vi "Define Test.vi"(8 "error in":errorcluster, 11 "Label (VI Title)":string) -> (0 "error out":errorcluster, 2 "Properties.Test":refnum<class "Properties.Test.lvclass">)   [LabVIEW 2021, in "Bananas.lvlib"]
uses:
  Bananas.lvlib
  <vilib>/addons/_JKI Toolkits/Caraya/classes/Properties.Test/Properties.Test.lvclass
  <vilib>/addons/_JKI Toolkits/Caraya/classes/Test/Test.lvclass
  Banana/Banana.lvclass
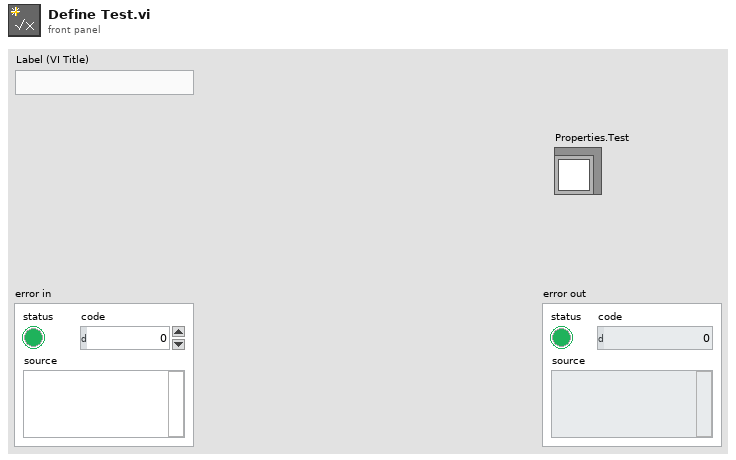
[diagram p1: front panel]
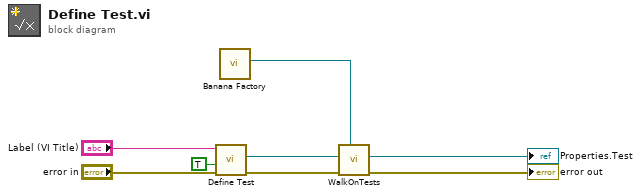
[diagram p0: block diagram]
diagram:
  n1 = call <vilib>:"Define Test.vi"("error in (no error)"="error in", "Register with caller (F)"=TRUE, "Label (VI Title)"="Label (VI Title)") -> ("error out"=w6:errorcluster, "Properties.Test"=w3:refnum<class "Properties.Test.lvclass">)  [unwired: 7 in]
  n2 = call "Banana Factory.vi"() -> ("Bunch"=w1:refnum<class "Banana.lvclass">)  [unwired: 11 in]
  n3 = call "WalkOnTests.vi"("Bunch"=w1, "error in (no error)"=w6, "Properties.Test"=w3) -> ("error out"=→"error out":errorcluster, "Properties.Test out"=→"Properties.Test":refnum<class "Properties.Test.lvclass">)  [unwired: 7 in]
